vi "Set Item Property (Dependent Node Pointer).vi"(8 "error in (no error)":errorcluster, 9 "Dependent Node Ref":T1=18446744073709551615 format="%.0x", 10 "Property Name":string, 11 "Item Ref in":T1 format="%.0x") -> (0 "error out":errorcluster, 3 "Item Ref out":T1 format="%.0x", 4 "Replaced":bool)   [LabVIEW 2020, in "Custom Device API.lvlib"]
doc: "Sets a <B>Property Name</B> and <B>Value</B> for an item property and saves this information in the system definition file. If the <B>Property Name</B> you specify already exists, this VI overwrites the property. Wire data to the <B>Value</B> input to determine the polymorphic instance to use or manually select the instance."
uses:
  <vilib>/NI VeriStand/Custom Device API/Custom Device API.lvlib
  <vilib>/NI VeriStand/Custom Device API/Custom Device Item Ref.ctl
  ed612387-504b-45df-9223-067018ed7dad.vi
  <vilib>/NI VeriStand/Custom Device API/Custom Device Offline Path.vi
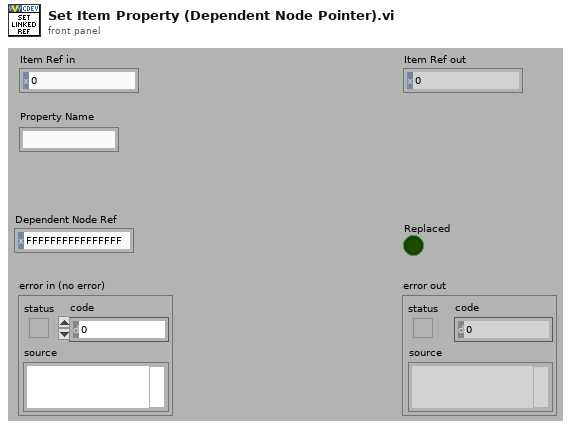
[diagram p1: front panel]
types:
  T1 = typedef "Custom Device API.lvlib/Custom Device Item Ref.ctl" = u64
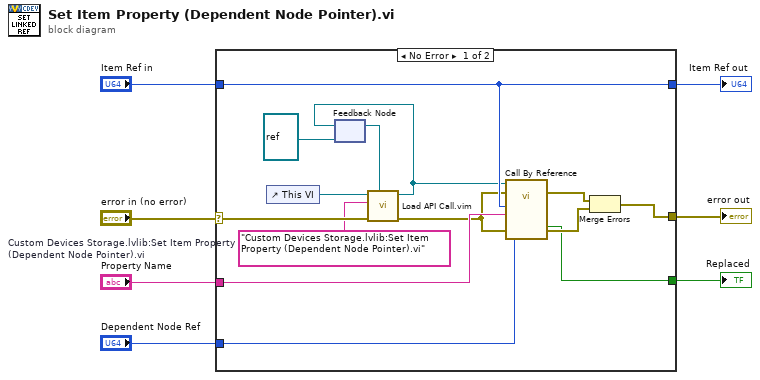
[diagram p0: block diagram]
diagram:
  n1 = case shown="No Error" "error in (no error)" {
    selector: "error in (no error)" -> [w13 w23]
    tunnel: "Item Ref in" -> [w16 w22]
    tunnel: [w16 w22] -> w6
    tunnel: [w20 w23] -> w5
    tunnel: "Property Name" -> [w19 _]
    tunnel: [w18 _] -> w3
    tunnel: "Dependent Node Ref" -> [w17 _]
    frame No Error {
      w9 = "Custom Devices Storage.lvlib:Set Item Property (Dependent Node Pointer).vi"  # Custom Devices Storage.lvlib:Set Item Property (Dependent Node Pointer).vi
      n2 = control-ref of="This VI"() -> (w14:refnum<vi>)
      n3 = feedback #1(refnum<vi> refnum ("type specifier VI Refnum (for type only)")) -> (w15:refnum<vi>)
      n4 = call "Load API Call.vim"("VI reference in"=w15, "error in (no error)"=w13, "VI qualified name"=w9, "Caller VI ref"=w14) -> ("error out"=w12:errorcluster, "VI reference"=w11:refnum<vi>)  [unwired: 6 in]
      n5 = feedback-in #1(w11) -> ()
      n6 = call-by-ref "?"(reference=w11, error in=w12, 8:"error in (no error)"=w12, "Dependent Node"=w17, "Property Name"=w19, "Item Ref in"=w16) -> (error out=w8:errorcluster, 0:"error out"=w21:errorcluster, "Replaced"=w18:bool)  [unwired: 5 in, 2 out]
      n7 = Merge Errors(w8, w21) -> (w20:errorcluster)
    }
    frame Error {
    }
  }
  "Item Ref out" <- w6
  "error out" <- w5
  "Replaced" <- w3
